vi "distanceRobotToBall.vi"(8 "error in (no error)":errorcluster, 9 "Robot":refnum<class "Robot.lvclass">, 10 "Ball":refnum<class "Ball.lvclass">, 11 "Utilities in":refnum<class "Utilities.lvclass">) -> (0 "error out":errorcluster, 2 "Distance Robot To Ball":dbl, 3 "Utilities out":refnum<class "Utilities.lvclass">)   [LabVIEW 2023, in "Utilities.lvclass"]
uses:
  Utilities.lvclass
  Robot_class/Robot.lvclass
  C:/Users/roboi/Downloads/VSS_AI-Larc2023 - Copia (2)/Object_class/Object.lvclass
  Ball_class/Ball.lvclass
  Object_class/Object.lvclass/Object.ctl
  Object_class/Read x.vi
  Object_class/Read y.vi
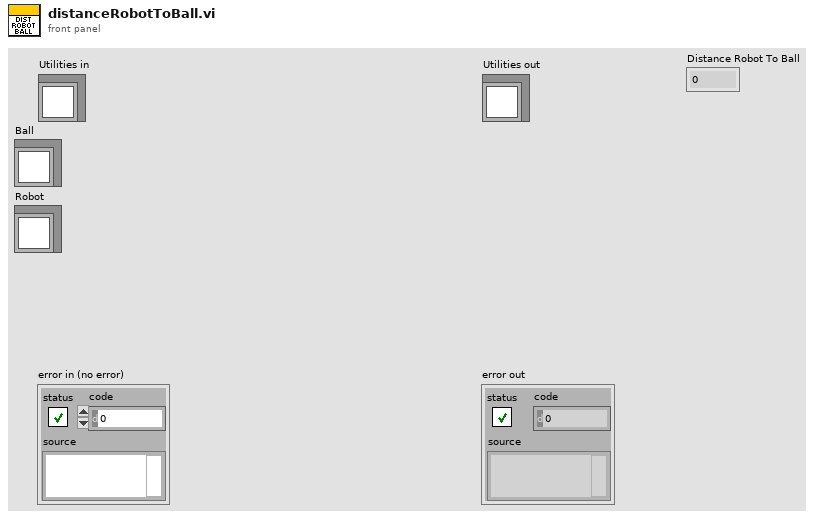
[diagram p1: front panel]
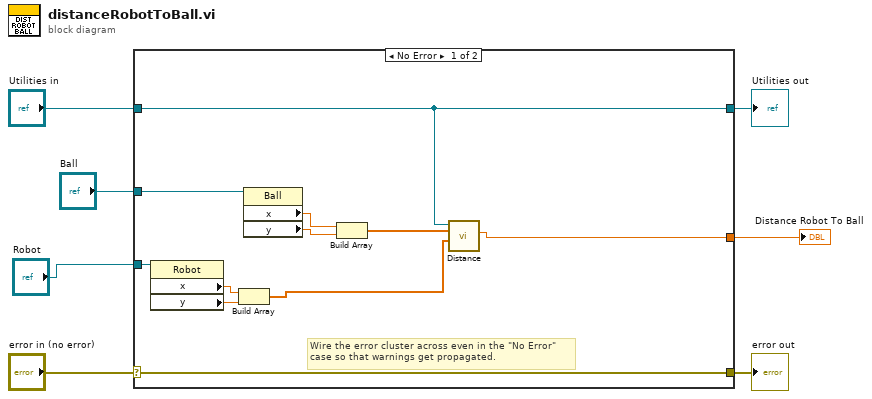
[diagram p0: block diagram]
diagram:
  n1 = case shown="No Error" "error in (no error)" {
    selector: "error in (no error)" -> [w18 w20]
    tunnel: [w18 w20] -> w6
    tunnel: [w10 w19] -> w4
    tunnel: "Utilities in" -> [w10 w19]
    tunnel: "Robot" -> [w17 _]
    tunnel: [w9 _] -> w2
    tunnel: "Ball" -> [w8 _]
    frame No Error {
      # "Wire the error cluster across even in the \"No Error\"\ncase so that warnings get propagated."
      n2 = property class="Robot"(reference=w17) -> ("x"=w16:dbl, "y"=w15:dbl)  [unwired: 1 in, 2 out]
      n3 = Build Array(w16, w15) -> (w11:dbl[])
      n4 = property class="Ball"(reference=w8) -> ("x"=w14:dbl, "y"=w13:dbl)  [unwired: 1 in, 2 out]
      n5 = Build Array(w14, w13) -> (w12:dbl[])
      n6 = call "Distance.vi"("P1"=w11, "P2"=w12, "Utilities in"=w10) -> ("Distance"=w9:dbl)  [unwired: 6 in, 2 out]
    }
    frame Error {
    }
  }
  "error out" <- w6
  "Utilities out" <- w4
  "Distance Robot To Ball" <- w2
